vi "GDSLvIcon_CalcWordsPerRow.vi"(1 "Max nr of rows":i32, 2 "Pixel width":i32, 3 "wordData":T1[](array[typedef]), 4 "words":string[](array[string]), 5 "error in (no error)":errorcluster) -> (12 "wordData out":T1[](array[typedef]), 15 "CompressRow":bool[](array[boolean]), 16 "WordsPerRow":i32[](array[numeric]), 17 "NoOfRowsRequired":i32, 19 "error out":errorcluster)   [LabVIEW 2020]
uses:
  GDSLvIcon_WordDataType.ctl
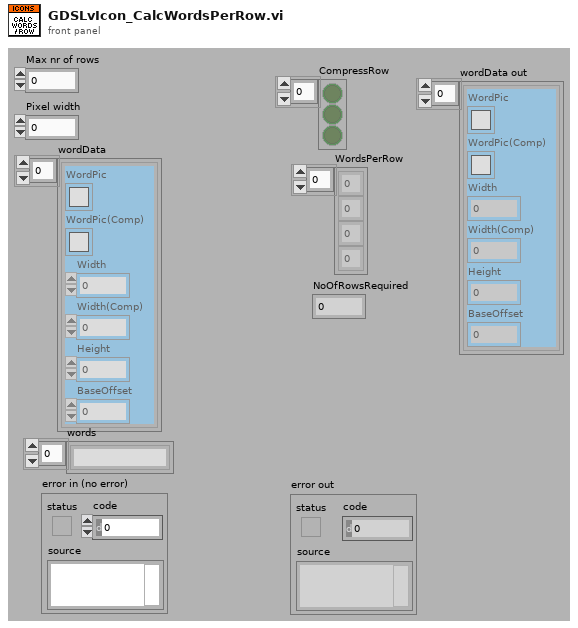
[diagram p1: front panel]
types:
  T1 = typedef "GDSLvIcon_WordDataType.ctl" = cluster{"WordPic":bool[][], "WordPic(Comp)":bool[][], "Width":i32, "Width(Comp)":i32, "Height":i32, "BaseOffset":i32}
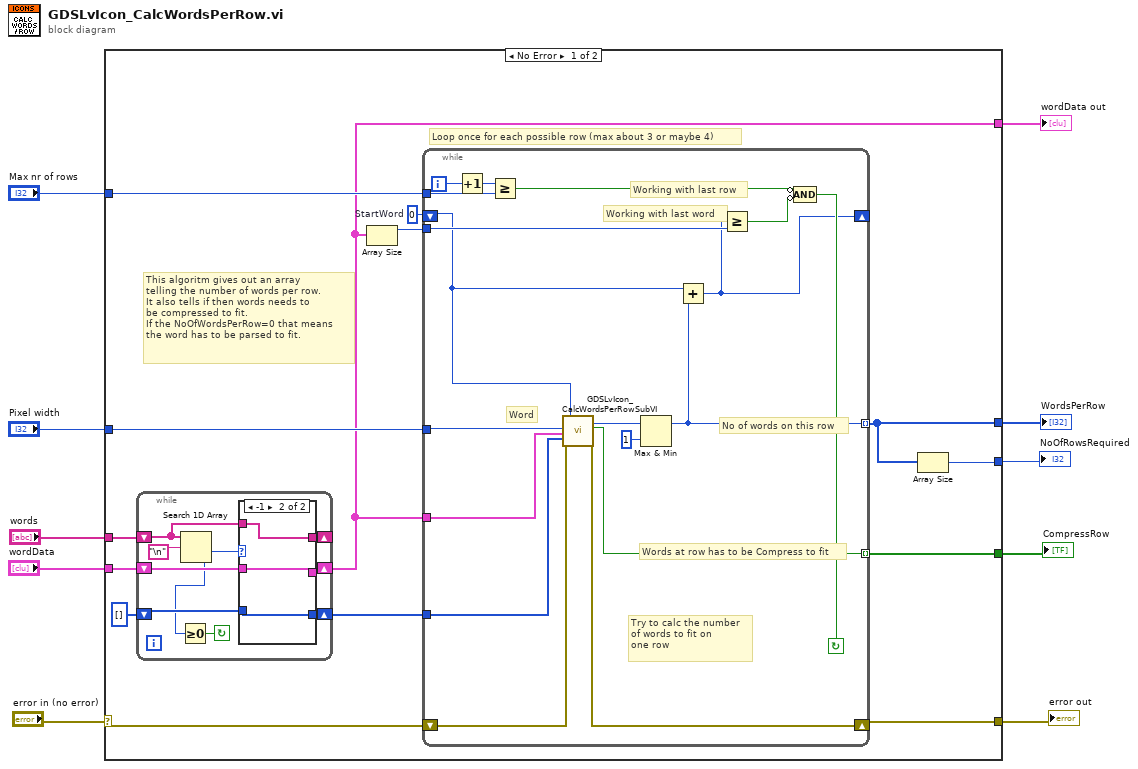
[diagram p0: block diagram]
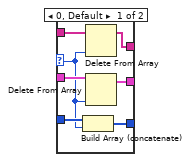
[diagram p2: hidden frame]
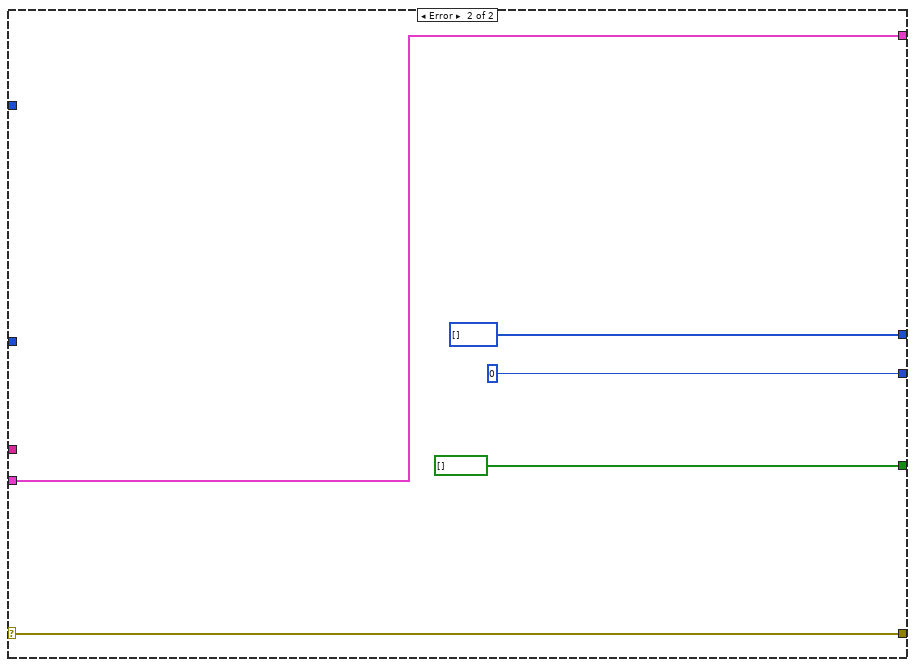
[diagram p3: hidden frame]
diagram:
  n1 = case shown="No Error" "error in (no error)" {
    selector: "error in (no error)" -> [w11 w66]
    tunnel: "Pixel width" -> [w24 _]
    tunnel: "Max nr of rows" -> [w23 _]
    tunnel: [w20 0] -> w8
    tunnel: [w19 bool[] []] -> w7
    tunnel: "words" -> [w17 _]
    tunnel: "wordData" -> [w16 w65]
    tunnel: [w15 w65] -> w4
    tunnel: [w14 i32[] []] -> w3
    tunnel: [w12 w66] -> w1
    frame No Error {
      w22 = 0  # StartWord
      # "This algoritm gives out an array\ntelling the number of words per row.\nIt also tells if then words needs to\nbe compressed to fit.\nIf the NoOfWordsPerRow=0 that means\nthe word has to be parsed to fit."
      # "Loop once for each possible row (max about 3 or maybe 4)"
      n2 = while {
        shift-left: i32[] [] -> [w46]
        shift-right: [w45] -> w13
        shift-left: w17 -> [w48]
        shift-right: [w47] -> _
        shift-left: w16 -> [w50]
        shift-right: [w49] -> w15
        stop <- w43 continue-if-true
        n3 = Search 1D Array(1D array=w48, element="\n") -> (index of element=w44:i32)  [unwired: 1 in]
        n4 = Greater Or Equal To 0?(x=w44) -> (x >= 0?=w43:bool)
        n5 = case shown="-1" w44 {
          selector: w44 -> [w53 _]
          tunnel: w50 -> [w58 w60]
          tunnel: [w57 w60] -> w49
          tunnel: w48 -> [w56 w61]
          tunnel: [w55 w61] -> w47
          tunnel: w46 -> [w54 w59]
          tunnel: [w52 w59] -> w45
          frame 0, Default {
            n6 = Build Array (concatenate)(w54, w53) -> (w52:i32[])
            n7 = Delete From Array(array=w56, index=w53) -> (array with subset deleted=w55:string[])  [unwired: 1 in, 1 out]
            n8 = Delete From Array(array=w58, index=w53) -> (array with subset deleted=w57:T1[])  [unwired: 1 in, 1 out]
          }
          frame -1 {
          }
        }
      }
      n9 = Array Size(array=w15) -> (size(s)=w21:i32)
      n10 = while {
        shift-left: w11 -> [w29]
        shift-right: [w30] -> w12
        tunnel: w13 -> [w31]
        tunnel: [w34] -> w19 mode=indexing
        tunnel: [w25] -> w14 mode=indexing
        tunnel: w21 -> [w36]
        shift-left: w22 -> [w33]
        shift-right: [w28] -> _
        tunnel: w24 -> [w35]
        tunnel: w15 -> [w32]
        tunnel: w23 -> [w41]
        i -> [w38]
        stop <- w39 continue-if-true
        # "Word"
        # "Try to calc the number \nof words to fit on \none row"
        # "No of words on this row"
        # "Words at row has to be Compress to fit"
        # "Working with last row"
        # "Working with last word"
        n11 = Increment(x=w38) -> (x+1=w42:i32)
        n12 = Greater Or Equal?(x=w42, y=w41) -> (x >= y?=w40:bool)
        n13 = call "GDSLvIcon_CalcWordsPerRowSubVI.vi"("Pixel width"=w35, "wordData"=w32, "EnterCharAtTheseLocations"=w31, "error in (no error)"=w29, "StartWordIndex"=w33) -> ("Words"=w26:i32, "RowNeedsToBeCompressed"=w34:bool, "error out"=w30:errorcluster)  [unwired: 12 in]
        n14 = Max & Min(x=w26, y=1) -> (max(x,y)=w25:i32)  [unwired: 1 out]
        n15 = Add(x=w33, y=w25) -> (x+y=w28:i32)
        n16 = Greater Or Equal?(x=w28, y=w36) -> (x >= y?=w37:bool)
        n17 = Compound Arithmetic op=AND(invert w40, invert w37) -> (w39:bool)
      }
      n18 = Array Size(array=w14) -> (size(s)=w20:i32)
    }
    frame Error {
    }
  }
  "WordsPerRow" <- w3
  "CompressRow" <- w7
  "error out" <- w1
  "NoOfRowsRequired" <- w8
  "wordData out" <- w4
